vi "Read IO List.vi"() -> ()   [LabVIEW 2011]
panel:
  out "String 2":string
  out "String":string
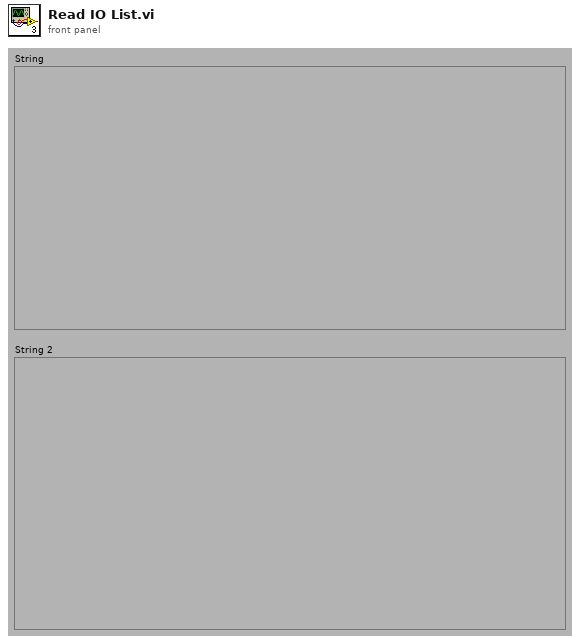
[diagram p1: front panel]
types:
  T1 = typedef "Fixed Analog Channel Definition.ctl" = cluster{"ID":u16, "Name":string, "Quantity":T2, "Unit":string, "Maximum upd":T3, "Comment":string, "Help file Name":string, "Help file Section ":string, "Category":T4, "User adjustable Scaling":bool, "Default Scaling":T5, "In use":bool, "Default Unit":i32}
  T2 = typedef "Quantity enum.ctl" = enum16{"Acceleration", "Angle", "Current", "Force", "Distance", "Pressure", "Resistance", "Rotational Speed", "Speed", "Temperature", "Tension", "Torque", "Voltage", "Weight"}
  T3 = typedef "Update frequensies.ctl" = enum16{"2 Hz", "1 Hz", "0.1 Hz"}
  T4 = typedef "Channel catagory Enum.ctl" = enum16{"No Category", "Power", "Temperature", "Pressure"}
  T5 = typedef "Scaling.ctl" = cluster{"Gain":dbl, "Offset":dbl}
  T6 = typedef "Fixed Digital Channel Definition.ctl" = cluster{"ID":u16, "Name":string, "NA Text":string, "Off Text":string, "On Text":string, "Maximum upd":T3, "Comment":string, "Help file Name":string, "Help file Section ":string, "Catagory":T4, "In use":bool}
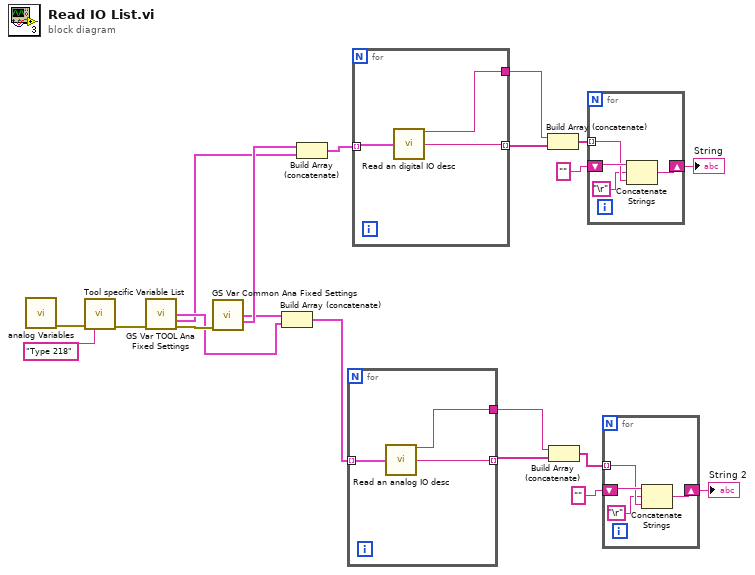
[diagram p0: block diagram]
diagram:
  n1 = call "analog Variables.vi"() -> ("error out"=w19:errorcluster)  [unwired: 15 in]
  n2 = call "Tool specific Variable List.vi"("error in (no error)"=w19, 12:"Type 218" ("Tool folder name")) -> ("error out"=w16:errorcluster)  [unwired: 13 in]
  n3 = call "GS Var TOOL Ana Fixed Settings.vi"("error in (no error)"=w16) -> ("Tool Analog var Fixed out"=w13:T1[], "Tool Digital Var Fixed out"=w11:T6[], "error out"=w15:errorcluster)  [unwired: 12 in]
  n4 = call "GS Var Common Ana Fixed Settings.vi"("error in (no error)"=w15) -> ("Common Analog Var Fixed out"=w17:T1[], "Common Digital var Fixed"=w18:T6[])  [unwired: 12 in, 1 out]
  n5 = Build Array (concatenate)(w17, w13) -> (w14:T1[])
  n6 = Build Array (concatenate)(w18, w11) -> (w12:T6[])
  n7 = for {
    tunnel: w14 -> [w23] mode=indexing
    tunnel: [w22] -> w10 mode=indexing
    tunnel: [w21] -> w9
    n8 = call "Read an analog IO desc.vi"("Variable Defenition"=w23) -> ("Header"=w21:string, "concatenated string"=w22:string)  [unwired: 13 in]
  }
  n9 = for {
    tunnel: w12 -> [w26] mode=indexing
    tunnel: [w25] -> w7
    tunnel: [w24] -> w8 mode=indexing
    n10 = call "Read an digital IO desc.vi"("Variable Defenition"=w26) -> ("Header"=w25:string, "concatenated string"=w24:string)  [unwired: 13 in]
  }
  n11 = Build Array (concatenate)(w7, w8) -> (w6:string[])
  n12 = Build Array (concatenate)(w9, w10) -> (w3:string[])
  n13 = for {
    tunnel: w6 -> [w28] mode=indexing
    shift-right: [w29] -> w2
    shift-left: "" -> [w30]
    n14 = Concatenate Strings(w30, "\r", w28) -> (w29:string)
  }
  "String" <- w2
  n15 = for {
    tunnel: w3 -> [w32] mode=indexing
    shift-right: [w33] -> w1
    shift-left: "" -> [w34]
    n16 = Concatenate Strings(w34, "\r", w32) -> (w33:string)
  }
  "String 2" <- w1
